vi "BlobTracking.vi"(0 "Image in":T1 {"Dialogs" format="%.0b"}, 1 "Init?":bool, 2 "K":dbl(slide)=0.49999999999999994 scale=0.0..1.0, 3 "Dimension":i32=20) -> (4 "lost track":bool, 5 "Image out":T1 {"Dialogs" format="%.0b"}, 6 "Predicted":cluster{"X":dbl, "Y":dbl}, 7 "Centroid":cluster{"X":dbl, "Y":dbl})   [LabVIEW 2024]
doc: "This VI will track a blob in a binary image. It returns the value of the predicted and determined (i.e. after testing analyzing a blob in the predicted region) centroid of the blob. By using this VI, your code does not have to do a blob analysis on the entire image. This is a more efficient method and therefore faster method of tracking objects in your images."
uses:
  <userlib>/ImageProcessing/QTLIB_2595_LV86/QT_Image.ctl
panel:
  out "Spot":cluster{"X":dbl, "Y":dbl}
  out "Start Centroid":cluster{"X":dbl, "Y":dbl}
  out "residual":cluster{"X":dbl, "Y":dbl}
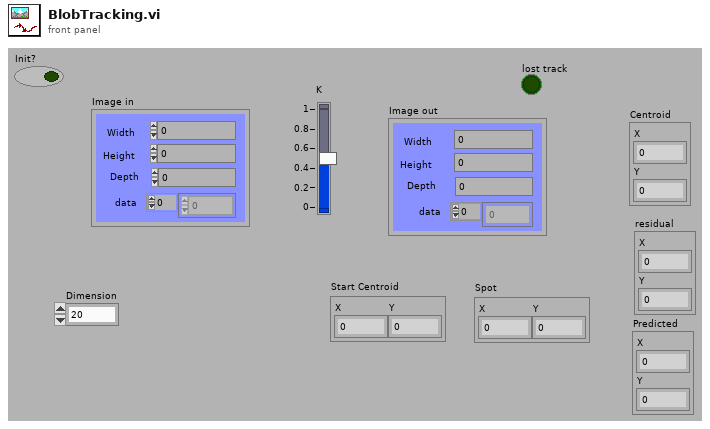
[diagram p1: front panel]
types:
  T1 = typedef "QT_Image.ctl" = cluster{"Width":i32, "Height":i32, "Depth":i32, "data":u8[], "Compressed data":u8[], "Color table":u32[], "Duration":i32, "Options":i32, "Timestamp":i32, "ID":i32, "Reserved":i32, "Dialogs":u32}
  T2 = cluster{"left":i16, "top":i16, "right":i16, "bottom":i16}
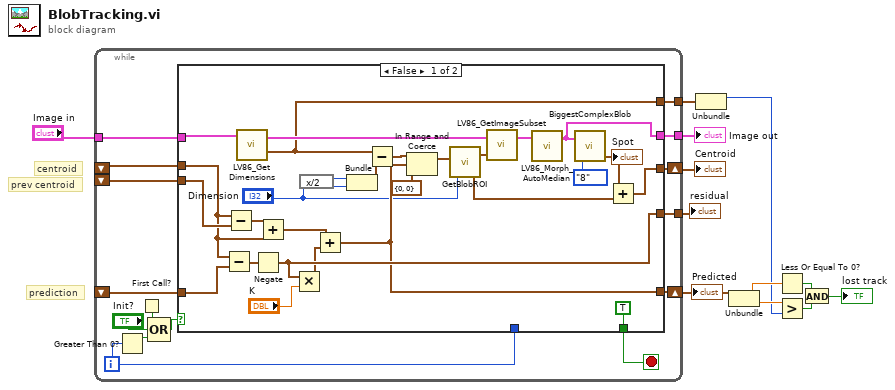
[diagram p0: block diagram]
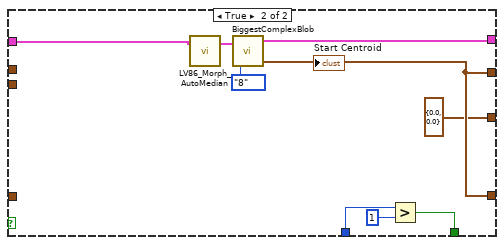
[diagram p2: hidden frame]
diagram:
  # "prediction"
  # "prev centroid"
  # "centroid"
  n1 = while {
    tunnel: "Image in" -> [w25]
    shift-right: [w27] -> w10
    shift-left: _ -> [w23]
    tunnel: [w26] -> w11
    shift-left: _ -> [w24]
    shift-right: [w21] -> w7
    shift-left: _ -> [w20]
    tunnel: [w19] -> w9
    tunnel: [w13] -> w4
    i -> [w18]
    stop <- w22 stop-if-true
    n2 = Greater Than 0?(x=w18) -> (x > 0?=w17:bool)
    n3 = First Call?() -> (First Call?: T/F=w14:bool)
    n4 = Compound Arithmetic op=OR(w14, "Init?", w17) -> (w15:bool)
    n5 = case shown="False" w15 {
      tunnel: [w48 w56] -> w27
      tunnel: [w29 w57] -> w26
      tunnel: w25 -> [w52 w58]
      tunnel: w24 -> [w44 _]
      tunnel: w23 -> [w39 _]
      tunnel: [TRUE w61] -> w22
      tunnel: w18 -> [_ w63]
      tunnel: [w35 w56] -> w21
      tunnel: w20 -> [w43 _]
      tunnel: [w41 cluster{"X":dbl, "Y":dbl} {"X"=0.0, "Y"=0.0} ("residual")] -> w19
      tunnel: [w31 _] -> w13
      frame False {
        n6 = Subtract(x=w39, y=w43) -> (x-y=w42:cluster{"X":dbl, "Y":dbl})
        n7 = Subtract(x=w39, y=w44) -> (x-y=w38:cluster{"X":dbl, "Y":dbl})
        n8 = call <userlib>:"LV86_Get Dimensions.vi"("Image In"=w52) -> ("Dimensions"=w31:cluster{"Width":i32, "Height":i32}, "Image Out"=w49:T1)  [unwired: 1 in]
        n9 = Negate(x=w42) -> (-x=w41:cluster{"X":dbl, "Y":dbl})
        n10 = Add(x=w38, y=w39) -> (x+y=w37:cluster{"X":dbl, "Y":dbl})
        n11 = Multiply(x=w41, y="K") -> (x*y=w36:cluster{"X":dbl, "Y":dbl})
        n12 = expression code="x/2"("Dimension") -> (w30:i32)
        n13 = Add(x=w37, y=w36) -> (x+y=w35:cluster{"X":dbl, "Y":dbl})
        n14 = Bundle("Dimension"=w30, "Dimension"=w30) -> (w32:cluster{"Dimension":i32, "Dimension":i32})  [unwired: 1 in]
        n15 = Subtract(x=w31, y=w32) -> (x-y=w33:cluster{i32, i32})
        n16 = In Range and Coerce(upper limit=w33, x=w35, lower limit=cluster{"right":i16, "bottom":i16} {"right"=0, "bottom"=0} ("upper limit")) -> (coerced(x)=w47:cluster{"X":dbl, "Y":dbl})  [unwired: 1 out]
        n17 = call <userlib>:"GetBlobROI.vi"("Dimension"="Dimension", "Centroid"=w47) -> ("Top Left"=w46:cluster{dbl, dbl}, "ROI"=w45:T2)
        n18 = call <userlib>:"LV86_GetImageSubset.vi"("ROI"=w45, "Image In"=w49) -> ("Image out"=w50:T1)  [unwired: 1 in]
        n19 = call <userlib>:"LV86_Morph_AutoMedian.vi"("Image in"=w50) -> ("Image out"=w29:T1)  [unwired: 2 in]
        n20 = call <userlib>:"BiggestComplexBlob.vi"("Connectivity"=enum16{"4", "8"}."8", "Image in"=w29) -> ("Centroid"=w53:cluster{"X":dbl, "Y":dbl})  [unwired: 2 out]
        "Spot" <- w53
        n21 = Add(x=w53, y=w46) -> (x+y=w48:cluster{dbl, dbl})
      }
      frame True {
        n22 = call <userlib>:"LV86_Morph_AutoMedian.vi"("Image in"=w58) -> ("Image out"=w59:T1)  [unwired: 2 in]
        n23 = call <userlib>:"BiggestComplexBlob.vi"("Connectivity"=enum16{"4", "8"}."8", "Image in"=w59) -> ("Centroid"=w56:cluster{"X":dbl, "Y":dbl}, "Image out"=w57:T1)  [unwired: 1 out]
        "Start Centroid" <- w56
        n24 = Greater?(x=w63, y=1) -> (0:w61:bool)
      }
    }
  }
  "Image out" <- w11
  "Centroid" <- w10
  "residual" <- w9
  "Predicted" <- w7
  n25 = Unbundle(w4) -> ("Width"=w3:i32)  [unwired: 1 out]
  n26 = Unbundle(w7) -> ("X"=w6:dbl, "Y"=w5:dbl)
  n27 = Less Or Equal To 0?(x=w6) -> (x <= 0?=w2:bool)
  n28 = Greater?(x=w5, y=w3) -> (0:w1:bool)
  n29 = And(x=w2, y=w1) -> (x .and. y?=→"lost track":bool)
